vi "XY to 2D.vi"(8 "error in (no error)":errorcluster, 11 "XY-data":cluster{"X-array":dbl[], "Y-array":dbl[]}[](array[cluster]) {"Y-array" format="%.2p"; "X-array" format="%.2p"}) -> (0 "error out":errorcluster, 2 "X Array":dbl[](array[numeric]), 3 "2D Y Array":dbl[][](array[numeric]))   [LabVIEW 2016, in "xy_utilities.lvlib"]
doc: "Interpolate Array of <b>XY-Data</b> to <b>2D Y Array</b> and <b>X Array</b>"
uses:
  xy_utilities.lvlib
  subVIs/Interpolate (multiple).vi
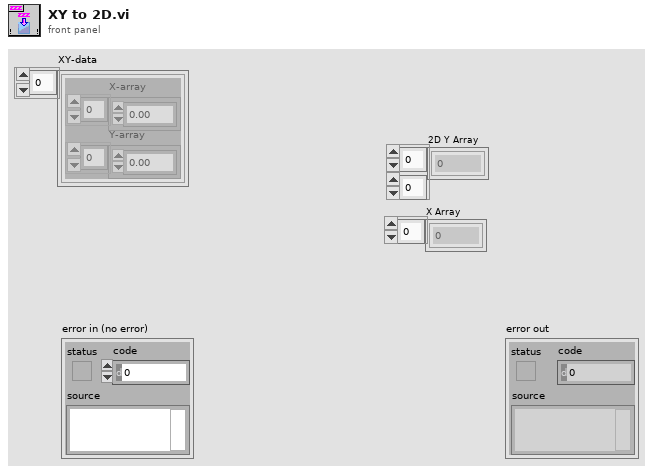
[diagram p1: front panel]
types:
  T1 = cluster{"X Low":dbl, "X High":dbl, "X Step":dbl, "Fake Point":dbl}
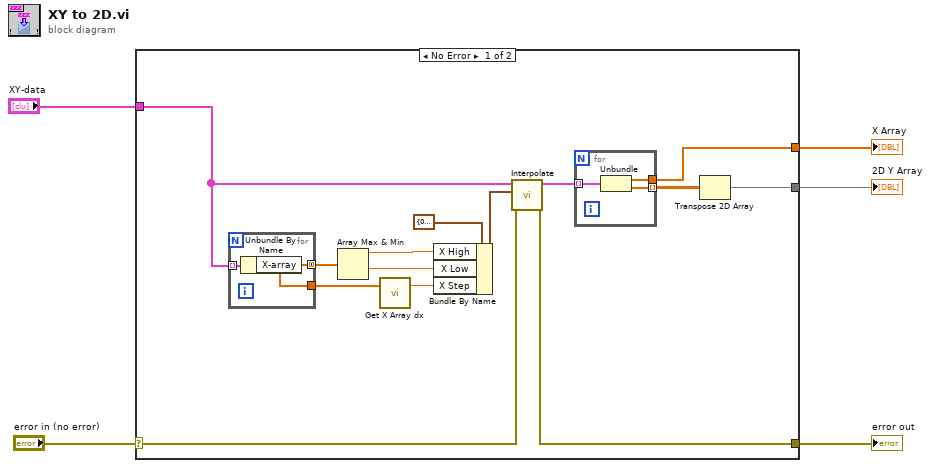
[diagram p0: block diagram]
diagram:
  n1 = case shown="No Error" "error in (no error)" {
    selector: "error in (no error)" -> [w10 w25]
    tunnel: [w9 w25] -> w4
    tunnel: "XY-data" -> [w11 _]
    tunnel: [w8 _] -> w2
    tunnel: [w7 _] -> w1
    frame No Error {
      n2 = for {
        tunnel: w11 -> [w21] mode=indexing
        tunnel: [w20] -> w14 mode=concatenating
        tunnel: [w20] -> w6
        n3 = Unbundle By Name(w21) -> ("X-array"=w20:dbl[])
      }
      n4 = Array Max & Min(array=w14) -> (max value=w17:dbl, min value=w18:dbl)  [unwired: 2 out]
      n5 = call "Get X Array dx.vi"("X-array"=w6) -> ("dX"=w13:dbl)  [unwired: 1 in, 1 out]
      n6 = Bundle By Name(cluster=T1 {"X Low"=0.05, "X High"=0.5, "X Step"=0.01, "Fake Point"=0.05} ("Configure"), "X High"=w17, "X Low"=w18, "X Step"=w13) -> (w16:T1)
      n7 = call-poly "Interpolate.vi"("error in (no error)"=w10, "Configure"=w16, "XY-data"=w11) -> ("error out"=w9:errorcluster, "Interpolated XY-data out"=w15:cluster{"X-array":dbl[], "Y-array":dbl[]}[])  [unwired: 7 in]
      n8 = for {
        tunnel: w15 -> [w24] mode=indexing
        tunnel: [w23] -> w12 mode=indexing
        tunnel: [w22] -> w7
        n9 = Unbundle(w24) -> ("X-array"=w22:dbl[], "Y-array"=w23:dbl[])
      }
      n10 = Transpose 2D Array(2D array=w12) -> (transposed array=w8:dbl[][])
    }
    frame Error {
    }
  }
  "error out" <- w4
  "2D Y Array" <- w2
  "X Array" <- w1
